vi "Read Status.vi"(8 "error in (no error)":errorcluster, 11 "SolarShutt in":refnum<class "SolarShutt.lvclass">) -> (0 "error out":errorcluster, 2 "Status":bool, 3 "SolarShutt out":refnum<class "SolarShutt.lvclass">)   [LabVIEW 2016, in "SolarShutt.lvclass"]
uses:
  SolarShutt.lvclass
  Shutter.lvclass
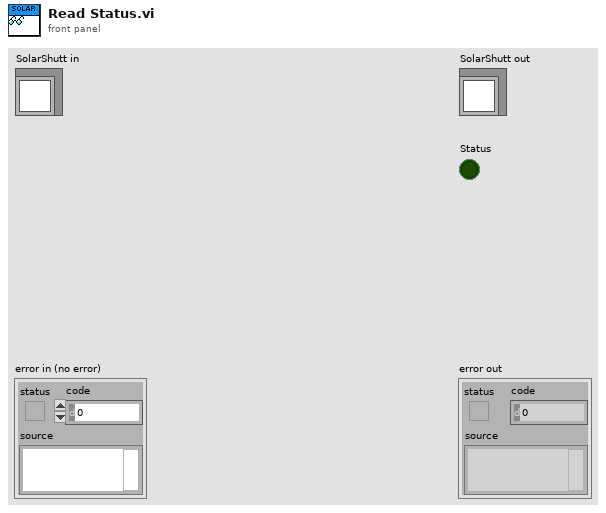
[diagram p1: front panel]
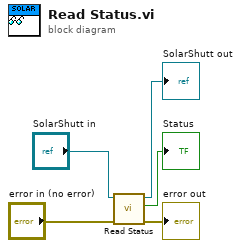
[diagram p0: block diagram]
diagram:
  n1 = call-parent "Read Status.vi"("error in (no error)"="error in (no error)", "Shutter in"="SolarShutt in") -> ("error out"=→"error out":errorcluster, "Status"=→"Status":bool, "Shutter out"=→"SolarShutt out":refnum<class "SolarShutt.lvclass">)  [unwired: 7 in]
